vi "Get Class Default Object.vi"(8 "error in (no error)":errorcluster, 9 "Library Path/Name":string, 10 "Class Path/Name":string, 11 "CS++Factory in":refnum<class "CS++Factory.lvclass">) -> (0 "error out":errorcluster, 2 "Class Default Object":refnum<class>, 3 "CS++Factory out":refnum<class "CS++Factory.lvclass">)   [LabVIEW 2013, in "CS++BaseClasses.lvlib" / "CS++Factory.lvclass"]
doc: "This is a dynamic dispatch VI.\n\n It is used to return an object with LabVIEW class default value. It becomed loaded from disk using <b>Class</b> as path. If the class is not found or an error is generated it ti tried to return a class default object from memory. \n\nThis helps testing classes during development and building application with statically linked classes with all dependencies.\n\nDerived classes can override this VI in order to load classes into memory as plugin, e.g. precompiled lvlibs."
uses:
  CS++Factory.lvclass
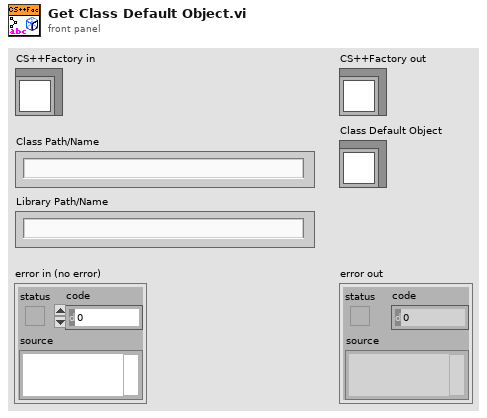
[diagram p1: front panel]
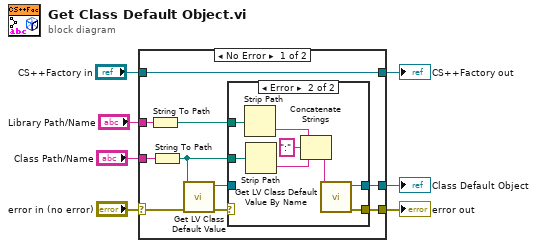
[diagram p0: block diagram]
diagram:
  n1 = case shown="No Error" "error in (no error)" {
    selector: "error in (no error)" -> [w15 w29]
    tunnel: [w10 w29] -> w6
    tunnel: [w17 w28] -> w4
    tunnel: "CS++Factory in" -> [w17 w28]
    tunnel: "Class Path/Name" -> [w16 _]
    tunnel: [w13 _] -> w2
    tunnel: "Library Path/Name" -> [w9 _]
    frame No Error {
      n2 = String To Path(string=w9) -> (path=w8:path)
      n3 = String To Path(string=w16) -> (path=w11:path)
      n4 = call <vilib>:"Get LV Class Default Value.vi"("error in (no error)"=w15, "class path"=w11) -> ("error out"=w14:errorcluster, "object"=w12:refnum<class>)  [unwired: 8 in]
      n5 = case shown="Error" w14 {
        selector: w14 -> [w18 _]
        tunnel: [w19 w25] -> w13
        tunnel: w12 -> [w19 _]
        tunnel: w11 -> [_ w26]
        tunnel: [w18 w24] -> w10
        tunnel: w8 -> [_ w23]
        frame No Error {
        }
        frame Error {
          n6 = Strip Path(path=w23) -> (name=w21:string)  [unwired: 1 out]
          n7 = Strip Path(path=w26) -> (name=w27:string)  [unwired: 1 out]
          n8 = Concatenate Strings(w21, ":" ("string"), w27) -> (w22:string)
          n9 = call <vilib>:"Get LV Class Default Value By Name.vi"("class name"=w22) -> ("error out"=w24:errorcluster, "object"=w25:refnum<class>)  [unwired: 9 in]
        }
      }
    }
    frame Error {
    }
  }
  "error out" <- w6
  "CS++Factory out" <- w4
  "Class Default Object" <- w2
